vi "Washer ERD List.vi"(7 "Enable Diagnostic Data":T1, 8 "Error In":errorcluster, 11 "Disable ERD (Main)":bool) -> (0 "Error Out":errorcluster, 2 "Header Array":string[](array[string]), 3 "Read ERD List":T2[](array[typedef]) {"ERD Number" format="%.0x"})   [LabVIEW 2016]
uses:
  type defs/ERD Read Data In.ctl
  type defs/Data Type.ctl
  Washer HCC/Washer HCC NEWFI/Type Definitions/HCC Washer Types.ctl
  library/GEA2_Toolkit.lvlib
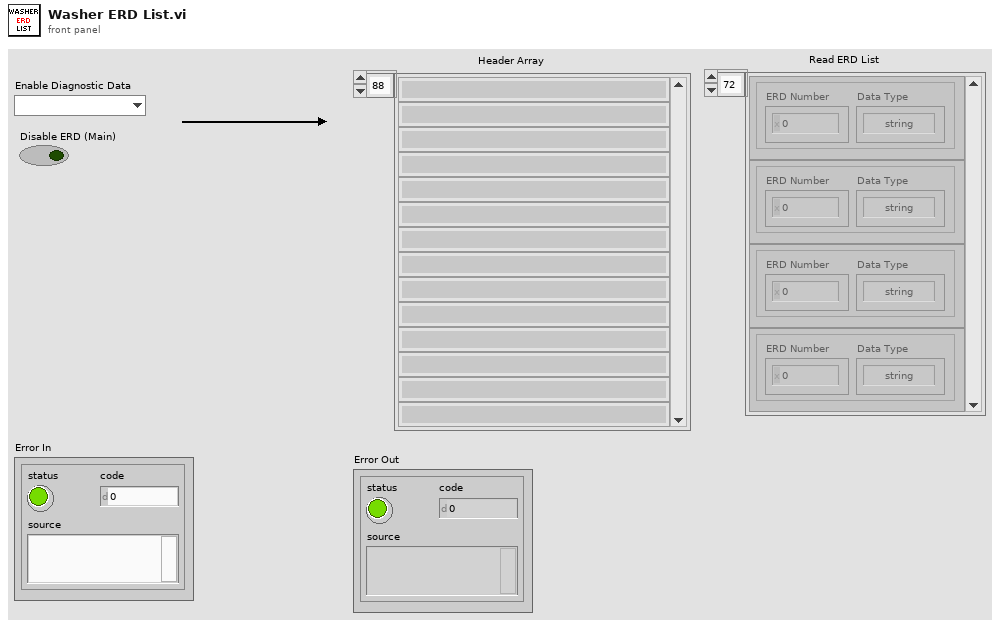
[diagram p1: front panel]
types:
  T1 = typedef "HCC Washer Types.ctl" = enum16{"", "Viper Washer", "Hawk Washer", "2015 Washer", "2017 Washer"}
  T2 = typedef "GEA2_Toolkit.lvlib/ERD Read Data In.ctl" = cluster{"ERD Number":u16, "Data Type":T3}
  T3 = typedef "GEA2_Toolkit.lvlib/Data Type.ctl" = enum16{"string", "boolean", "uint8_t", "uint16_t", "uint32_t", "uint64_t"}
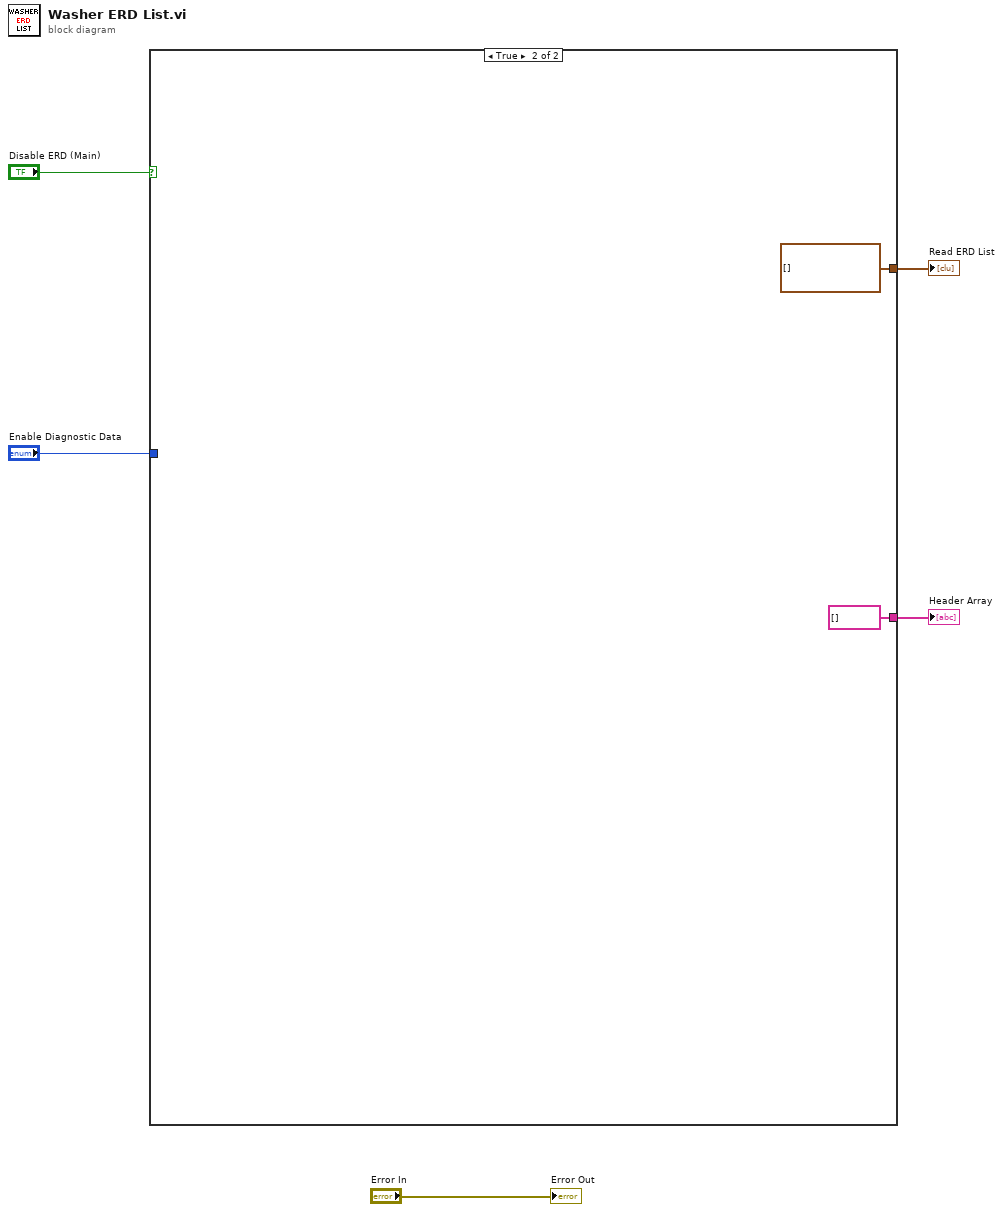
[diagram p0: block diagram]
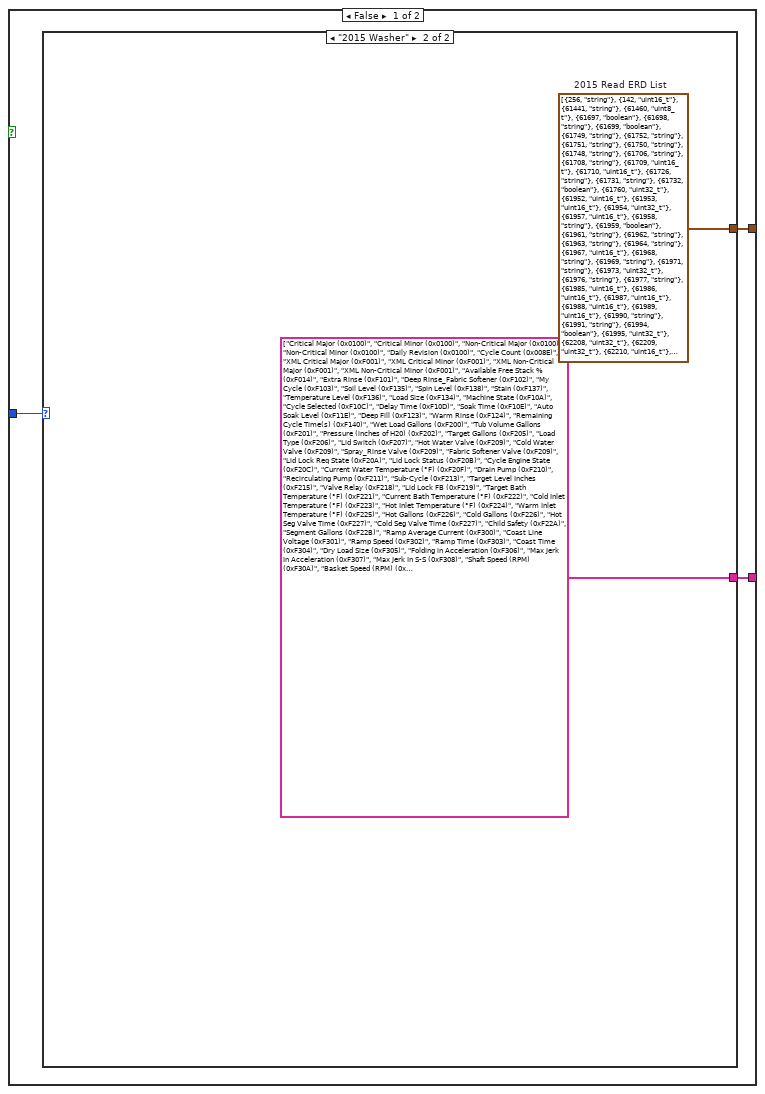
[diagram p2: hidden frame]
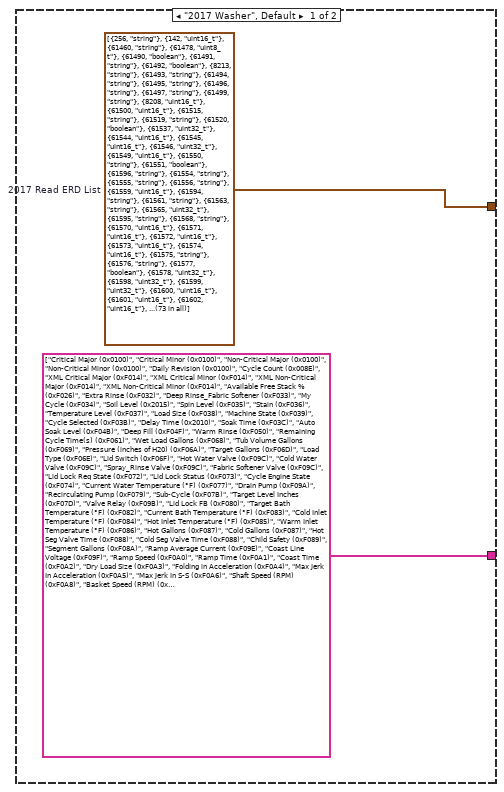
[diagram p3: hidden frame]
diagram:
  n1 = case shown="True" "Disable ERD (Main)" {
    tunnel: [w8 string[] []] -> w3
    tunnel: [w7 T2[] [] ("Read ERD List")] -> w4
    tunnel: "Enable Diagnostic Data" -> [w6 _]
    frame False {
      n2 = case shown="\"2015 Washer\"" w6 {
        tunnel: [string[] ["Critical Major (0x0100)", "Critical Minor (0x0100)", "Non-Critical Major (0x0100)", "Non-Critical Minor (0x0100)", "Daily Revision (0x0100)", "Cycle Count (0x008E)", "XML Critical Major (0xF014)", "XML Critical Minor (0xF014)", "XML Non-Critical Major (0xF014)", "XML Non-Critical Minor (0xF014)", "Available Free Stack % (0xF026)", "Extra Rinse (0xF032)", "Deep Rinse_Fabric Softener (0xF033)", "My Cycle (0xF034)", "Soil Level (0x2015)", "Spin Level (0xF035)", "Stain (0xF036)", "Temperature Level (0xF037)", "Load Size (0xF038)", "Machine State (0xF039)", "Cycle Selected (0xF03B)", "Delay Time (0x2010)", "Soak Time (0xF03C)", "Auto Soak Level (0xF04B)", "Deep Fill (0xF04F)", "Warm Rinse (0xF050)", "Remaining Cycle Time(s) (0xF061)", "Wet Load Gallons (0xF068)", "Tub Volume Gallons (0xF069)", "Pressure (inches of H20) (0xF06A)", "Target Gallons (0xF06D)", "Load Type (0xF06E)", "Lid Switch (0xF06F)", "Hot Water Valve (0xF09C)", "Cold Water Valve (0xF09C)", "Spray_Rinse Valve (0xF09C)", "Fabric Softener Valve (0xF09C)", "Lid Lock Req State (0xF072)", "Lid Lock Status (0xF073)", "Cycle Engine State (0xF074)", "Current Water Temperature (°F) (0xF077)", "Drain Pump (0xF09A)", "Recirculating Pump (0xF079)", "Sub-Cycle (0xF07B)", "Target Level Inches (0xF07D)", "Valve Relay (0xF09B)", "Lid Lock FB (0xF080)", "Target Bath Temperature (°F) (0xF082)", "Current Bath Temperature (°F) (0xF083)", "Cold Inlet Temperature (°F) (0xF084)", "Hot Inlet Temperature (°F) (0xF085)", "Warm Inlet Temperature (°F) (0xF086)", "Hot Gallons (0xF087)", "Cold Gallons (0xF087)", "Hot Seg Valve Time (0xF088)", "Cold Seg Valve Time (0xF088)", "Child Safety (0xF089)", "Segment Gallons (0xF08A)", "Ramp Average Current (0xF09E)", "Coast Line Voltage (0xF09F)", "Ramp Speed (0xF0A0)", "Ramp Time (0xF0A1)", "Coast Time (0xF0A2)", "Dry Load Size (0xF0A3)", "Folding in Acceleration (0xF0A4)", "Max Jerk In Acceleration (0xF0A5)", "Max Jerk In S-S (0xF0A6)", "Shaft Speed (RPM) (0xF0A8)", "Basket Speed (RPM) (0xF0A9)", "Current RMS (Amps) (0xF0AB)", "Target Speed (RPM) (0xF0AC)", "Motor Mode (0xF0B1)", "OOB Detected in Acceleration (0xF0B3)", "OOB Detected in S-S (0xF0B4)", "OOB ReDistribution Required (0xF0B5)", "Motor Profile Status (0xF0B7)", "Motor Profile (0xF0B7)", "Mode Shift Status (0xFF22)", "ME Relay (0xF0BE)", "Mode Shift FB (0xF0BF)", "MS Motor (0xF0C0)", "Partial Coast Time (0xF0C6)", "Ramp Line Voltage (0xF0C7)", "Personality (0xFF00)", "Reset Source (0xFF02)", "DC Bus Voltage RMS value (0xF0C4)"] string[] ["Critical Major (0x0100)", "Critical Minor (0x0100)", "Non-Critical Major (0x0100)", "Non-Critical Minor (0x0100)", "Daily Revision (0x0100)", "Cycle Count (0x008E)", "XML Critical Major (0xF001)", "XML Critical Minor (0xF001)", "XML Non-Critical Major (0xF001)", "XML Non-Critical Minor (0xF001)", "Available Free Stack % (0xF014)", "Extra Rinse (0xF101)", "Deep Rinse_Fabric Softener (0xF102)", "My Cycle (0xF103)", "Soil Level (0xF135)", "Spin Level (0xF138)", "Stain (0xF137)", "Temperature Level (0xF136)", "Load Size (0xF134)", "Machine State (0xF10A)", "Cycle Selected (0xF10C)", "Delay Time (0xF10D)", "Soak Time (0xF10E)", "Auto Soak Level (0xF11E)", "Deep Fill (0xF123)", "Warm Rinse (0xF124)", "Remaining Cycle Time(s) (0xF140)", "Wet Load Gallons (0xF200)", "Tub Volume Gallons (0xF201)", "Pressure (inches of H20) (0xF202)", "Target Gallons (0xF205)", "Load Type (0xF206)", "Lid Switch (0xF207)", "Hot Water Valve (0xF209)", "Cold Water Valve (0xF209)", "Spray_Rinse Valve (0xF209)", "Fabric Softener Valve (0xF209)", "Lid Lock Req State (0xF20A)", "Lid Lock Status (0xF20B)", "Cycle Engine State (0xF20C)", "Current Water Temperature (°F) (0xF20F)", "Drain Pump (0xF210)", "Recirculating Pump (0xF211)", "Sub-Cycle (0xF213)", "Target Level Inches (0xF215)", "Valve Relay (0xF218)", "Lid Lock FB (0xF219)", "Target Bath Temperature (°F) (0xF221)", "Current Bath Temperature (°F) (0xF222)", "Cold Inlet Temperature (°F) (0xF223)", "Hot Inlet Temperature (°F) (0xF224)", "Warm Inlet Temperature (°F) (0xF225)", "Hot Gallons (0xF226)", "Cold Gallons (0xF226)", "Hot Seg Valve Time (0xF227)", "Cold Seg Valve Time (0xF227)", "Child Safety (0xF22A)", "Segment Gallons (0xF22B)", "Ramp Average Current (0xF300)", "Coast Line Voltage (0xF301)", "Ramp Speed (0xF302)", "Ramp Time (0xF303)", "Coast Time (0xF304)", "Dry Load Size (0xF305)", "Folding in Acceleration (0xF306)", "Max Jerk In Acceleration (0xF307)", "Max Jerk In S-S (0xF308)", "Shaft Speed (RPM) (0xF30A)", "Basket Speed (RPM) (0xF30B)", "Current RMS (Amps) (0xF30D)", "Target Speed (RPM) (0xF30E)", "Motor Mode (0xF313)", "OOB Detected in Acceleration (0xF315)", "OOB Detected in S-S (0xF316)", "OOB ReDistribution Required (0xF317)", "Motor Profile Status (0xF319)", "Motor Profile (0xF319)", "Mode Shift Status (0xF31D)", "ME Relay (0xF321)", "Mode Shift FB (0xF322)", "MS Motor (0xF323)", "Partial Coast Time (0xF32D)", "Ramp Line Voltage (0xF32E)", "Personality (0xF000)", "Reset Source (0xF017)", "DC Bus Voltage RMS value (F32A)"]] -> w8
        tunnel: [w10 w11] -> w7
        frame "2017 Washer", Default {
          w10 = T2[] [{"ERD Number"=256, "Data Type"=enum."string"}, {"ERD Number"=142, "Data Type"=enum."uint16_t"}, {"ERD Number"=61460, "Data Type"=enum."string"}, {"ERD Number"=61478, "Data Type"=enum."uint8_t"}, {"ERD Number"=61490, "Data Type"=enum."boolean"}, {"ERD Number"=61491, "Data Type"=enum."string"}, {"ERD Number"=61492, "Data Type"=enum."boolean"}, {"ERD Number"=8213, "Data Type"=enum."string"}, {"ERD Number"=61493, "Data Type"=enum."string"}, {"ERD Number"=61494, "Data Type"=enum."string"}, {"ERD Number"=61495, "Data Type"=enum."string"}, {"ERD Number"=61496, "Data Type"=enum."string"}, {"ERD Number"=61497, "Data Type"=enum."string"}, {"ERD Number"=61499, "Data Type"=enum."string"}, {"ERD Number"=8208, "Data Type"=enum."uint16_t"}, {"ERD Number"=61500, "Data Type"=enum."uint16_t"}, {"ERD Number"=61515, "Data Type"=enum."string"}, {"ERD Number"=61519, "Data Type"=enum."string"}, {"ERD Number"=61520, "Data Type"=enum."boolean"}, {"ERD Number"=61537, "Data Type"=enum."uint32_t"}, {"ERD Number"=61544, "Data Type"=enum."uint16_t"}, {"ERD Number"=61545, "Data Type"=enum."uint16_t"}, {"ERD Number"=61546, "Data Type"=enum."uint32_t"}, {"ERD Number"=61549, "Data Type"=enum."uint16_t"}, {"ERD Number"=61550, "Data Type"=enum."string"}, {"ERD Number"=61551, "Data Type"=enum."boolean"}, {"ERD Number"=61596, "Data Type"=enum."string"}, {"ERD Number"=61554, "Data Type"=enum."string"}, {"ERD Number"=61555, "Data Type"=enum."string"}, {"ERD Number"=61556, "Data Type"=enum."string"}, {"ERD Number"=61559, "Data Type"=enum."uint16_t"}, {"ERD Number"=61594, "Data Type"=enum."string"}, {"ERD Number"=61561, "Data Type"=enum."string"}, {"ERD Number"=61563, "Data Type"=enum."string"}, {"ERD Number"=61565, "Data Type"=enum."uint32_t"}, {"ERD Number"=61595, "Data Type"=enum."string"}, {"ERD Number"=61568, "Data Type"=enum."string"}, {"ERD Number"=61570, "Data Type"=enum."uint16_t"}, {"ERD Number"=61571, "Data Type"=enum."uint16_t"}, {"ERD Number"=61572, "Data Type"=enum."uint16_t"}, {"ERD Number"=61573, "Data Type"=enum."uint16_t"}, {"ERD Number"=61574, "Data Type"=enum."uint16_t"}, {"ERD Number"=61575, "Data Type"=enum."string"}, {"ERD Number"=61576, "Data Type"=enum."string"}, {"ERD Number"=61577, "Data Type"=enum."boolean"}, {"ERD Number"=61578, "Data Type"=enum."uint32_t"}, {"ERD Number"=61598, "Data Type"=enum."uint32_t"}, {"ERD Number"=61599, "Data Type"=enum."uint32_t"}, {"ERD Number"=61600, "Data Type"=enum."uint16_t"}, {"ERD Number"=61601, "Data Type"=enum."uint16_t"}, {"ERD Number"=61602, "Data Type"=enum."uint16_t"}, {"ERD Number"=61603, "Data Type"=enum."uint16_t"}, {"ERD Number"=61604, "Data Type"=enum."string"}, {"ERD Number"=61605, "Data Type"=enum."string"}, {"ERD Number"=61606, "Data Type"=enum."string"}, {"ERD Number"=61608, "Data Type"=enum."uint16_t"}, {"ERD Number"=61609, "Data Type"=enum."uint16_t"}, {"ERD Number"=61611, "Data Type"=enum."uint16_t"}, {"ERD Number"=61612, "Data Type"=enum."string"}, {"ERD Number"=61617, "Data Type"=enum."string"}, {"ERD Number"=61619, "Data Type"=enum."boolean"}, {"ERD Number"=61620, "Data Type"=enum."boolean"}, {"ERD Number"=61621, "Data Type"=enum."boolean"}, {"ERD Number"=61623, "Data Type"=enum."string"}, {"ERD Number"=65314, "Data Type"=enum."string"}, {"ERD Number"=61630, "Data Type"=enum."boolean"}, {"ERD Number"=61631, "Data Type"=enum."boolean"}, {"ERD Number"=61632, "Data Type"=enum."boolean"}, {"ERD Number"=61638, "Data Type"=enum."uint16_t"}, {"ERD Number"=61639, "Data Type"=enum."uint16_t"}, {"ERD Number"=65280, "Data Type"=enum."uint8_t"}, {"ERD Number"=65282, "Data Type"=enum."string"}, {"ERD Number"=61636, "Data Type"=enum."uint16_t"}]  # 2017 Read ERD List
        }
        frame "2015 Washer" {
          w11 = T2[] [{"ERD Number"=256, "Data Type"=enum."string"}, {"ERD Number"=142, "Data Type"=enum."uint16_t"}, {"ERD Number"=61441, "Data Type"=enum."string"}, {"ERD Number"=61460, "Data Type"=enum."uint8_t"}, {"ERD Number"=61697, "Data Type"=enum."boolean"}, {"ERD Number"=61698, "Data Type"=enum."string"}, {"ERD Number"=61699, "Data Type"=enum."boolean"}, {"ERD Number"=61749, "Data Type"=enum."string"}, {"ERD Number"=61752, "Data Type"=enum."string"}, {"ERD Number"=61751, "Data Type"=enum."string"}, {"ERD Number"=61750, "Data Type"=enum."string"}, {"ERD Number"=61748, "Data Type"=enum."string"}, {"ERD Number"=61706, "Data Type"=enum."string"}, {"ERD Number"=61708, "Data Type"=enum."string"}, {"ERD Number"=61709, "Data Type"=enum."uint16_t"}, {"ERD Number"=61710, "Data Type"=enum."uint16_t"}, {"ERD Number"=61726, "Data Type"=enum."string"}, {"ERD Number"=61731, "Data Type"=enum."string"}, {"ERD Number"=61732, "Data Type"=enum."boolean"}, {"ERD Number"=61760, "Data Type"=enum."uint32_t"}, {"ERD Number"=61952, "Data Type"=enum."uint16_t"}, {"ERD Number"=61953, "Data Type"=enum."uint16_t"}, {"ERD Number"=61954, "Data Type"=enum."uint32_t"}, {"ERD Number"=61957, "Data Type"=enum."uint16_t"}, {"ERD Number"=61958, "Data Type"=enum."string"}, {"ERD Number"=61959, "Data Type"=enum."boolean"}, {"ERD Number"=61961, "Data Type"=enum."string"}, {"ERD Number"=61962, "Data Type"=enum."string"}, {"ERD Number"=61963, "Data Type"=enum."string"}, {"ERD Number"=61964, "Data Type"=enum."string"}, {"ERD Number"=61967, "Data Type"=enum."uint16_t"}, {"ERD Number"=61968, "Data Type"=enum."string"}, {"ERD Number"=61969, "Data Type"=enum."string"}, {"ERD Number"=61971, "Data Type"=enum."string"}, {"ERD Number"=61973, "Data Type"=enum."uint32_t"}, {"ERD Number"=61976, "Data Type"=enum."string"}, {"ERD Number"=61977, "Data Type"=enum."string"}, {"ERD Number"=61985, "Data Type"=enum."uint16_t"}, {"ERD Number"=61986, "Data Type"=enum."uint16_t"}, {"ERD Number"=61987, "Data Type"=enum."uint16_t"}, {"ERD Number"=61988, "Data Type"=enum."uint16_t"}, {"ERD Number"=61989, "Data Type"=enum."uint16_t"}, {"ERD Number"=61990, "Data Type"=enum."string"}, {"ERD Number"=61991, "Data Type"=enum."string"}, {"ERD Number"=61994, "Data Type"=enum."boolean"}, {"ERD Number"=61995, "Data Type"=enum."uint32_t"}, {"ERD Number"=62208, "Data Type"=enum."uint32_t"}, {"ERD Number"=62209, "Data Type"=enum."uint32_t"}, {"ERD Number"=62210, "Data Type"=enum."uint16_t"}, {"ERD Number"=62211, "Data Type"=enum."uint16_t"}, {"ERD Number"=62212, "Data Type"=enum."uint16_t"}, {"ERD Number"=62213, "Data Type"=enum."uint16_t"}, {"ERD Number"=62214, "Data Type"=enum."string"}, {"ERD Number"=62215, "Data Type"=enum."string"}, {"ERD Number"=62216, "Data Type"=enum."string"}, {"ERD Number"=62218, "Data Type"=enum."uint16_t"}, {"ERD Number"=62219, "Data Type"=enum."uint16_t"}, {"ERD Number"=62221, "Data Type"=enum."uint16_t"}, {"ERD Number"=62222, "Data Type"=enum."string"}, {"ERD Number"=62227, "Data Type"=enum."string"}, {"ERD Number"=62229, "Data Type"=enum."boolean"}, {"ERD Number"=62230, "Data Type"=enum."boolean"}, {"ERD Number"=62231, "Data Type"=enum."boolean"}, {"ERD Number"=62233, "Data Type"=enum."string"}, {"ERD Number"=62237, "Data Type"=enum."string"}, {"ERD Number"=62241, "Data Type"=enum."boolean"}, {"ERD Number"=62242, "Data Type"=enum."boolean"}, {"ERD Number"=62243, "Data Type"=enum."boolean"}, {"ERD Number"=62253, "Data Type"=enum."uint16_t"}, {"ERD Number"=62254, "Data Type"=enum."uint16_t"}, {"ERD Number"=61440, "Data Type"=enum."uint8_t"}, {"ERD Number"=61463, "Data Type"=enum."string"}, {"ERD Number"=62250, "Data Type"=enum."uint16_t"}]  # 2015 Read ERD List
        }
      }
    }
    frame True {
    }
  }
  "Read ERD List" <- w4
  "Header Array" <- w3
  "Error Out" <- "Error In"
